vi "NanotecSMCPD.i attribute.vi"(0 "VI Refnum":refnum<vi>, 2 "CLASS.i attribute":T1, 3 "Action":T2(ring), 5 "error in (no error)":errorcluster) -> (14 "VI Refnum out":refnum<vi>, 16 "CLASS.i attribute out":T1, 19 "error out":errorcluster)   [LabVIEW 2014, in "NanotecSMCPD.lvlib"]
doc: "This is a so-called functional global variable. It manages the access to a global variable in a thread-safe way. \n\nHere the attribute data of all instances of THIS class are stored. This is done for performance reasons.\n\nThe indicator \"attribute out\" carries only valid data upon calling the function \"get data\"\n\nLicense Agreement for this software:\n\nCopyright (C)\nGesellschaft für Schwerionenforschung, GSI\nPlanckstr. 1\n64291 Darmstadt\nGermany\n\nContact: D.Beck@gsi.de \n\nThis program is free software; you can redistribute it and/or modify it under the terms of the GNU General Public License as published by the Free Software Foundation; either version 2 of the license, or (at your option) any later version.\n\nThis program is distributed in the hope that it will be useful, but WITHOUT ANY WARRANTY; without even the implied warranty of MERCHANTABILITY or FITNESS FOR A PARTICULAR PURPOSE. See the GNU General License for more details (http://www.gnu.org).\n\nGesellschaft für Schwerionenforschung, GSI\nPlanckstr. 1, 64291 Darmstadt, Germany\nFor all questions and ideas contact: M.Richter@gsi.de, H.Brand@gsi.de or D.Beck@gsi.de.\nLast update: 17-JUN-2004"
uses:
  NanotecSMCPD.lvlib
  NanotecSMCPD.i attribute.ctl
  CSCore/CSSystem/CoreDefs/CoreDefs.error_type.ctl
  CSCore/CSSystem/CoreLib/CoreLib.lvlib
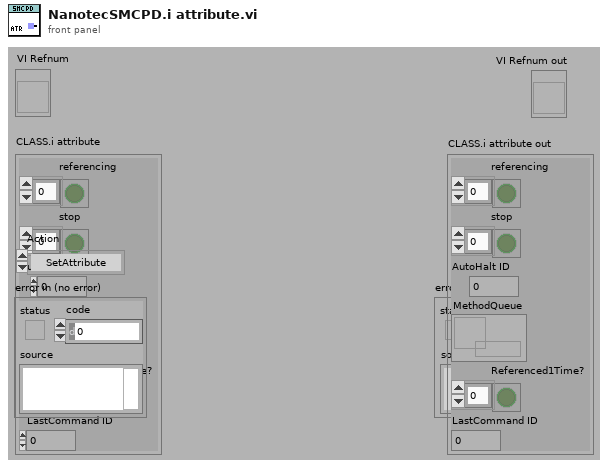
[diagram p1: front panel]
types:
  T1 = typedef "NanotecSMCPD.lvlib/NanotecSMCPD.i attribute.ctl" = cluster{"referencing":bool[], "stop":bool[], "AutoHalt ID":i32, "MethodQueue":refnum<queue>, "Referenced1Time?":bool[], "LastCommand ID":i32}
  T2 = enum16{"SetAttribute", "GetAttribute", "CreateAttribute", "DestroyAttribute", "DestroyAllAtributes"}
  T3 = typedef "CoreDefs.error_type.ctl" = enum16{"no error", "can't load process", "can't unload process", "process does not exist", "can't install process", "can't remove process", "unknown function", "time out", "can't execute function", "duplicate queue name", "super not found", "caller queue invalid", "can't ping process", "unknown error", "VISA Error", "VISA timeout", "GPIB timeout", "GPIB error", "communication error", "data type mismatch", "can't read data from OPC server", "can't write data to OPC server", "OET error", "function not implemented", "process already exists", "invalid Shared Variable name", "error writing Shared Variable", "error reading Shared Variable", "invalid client name", "corrupt database", "unknown class", "call not authorized", "parameter out of range", "OET timeout: can't get data to modify", "invalid queue name", "requested operation incompatible with current state", "event undefined", "event disabled", "state undefined", "caller is not a friend", "EventBuilder: bad eventID", "EventBuilder: no DAQ devices", "a thread must not stop itself", "UNUSED ELEMENT4", "DiscArchiver: eventData incomplete", "DiscArchiver: eventData does not belong to run", "DiscArchiver: can't open file", "DiscArchiver: can't write to file", "DiscArchiver: available disc space low", "can't acquire semaphore", "error reading data from database", "notifier object is not existing", "can't register process", "can't unregister process", "illegal event type", "object disabled", "object already exists", "can't change state", "Instrument not found", "no connection to remote node", "invalid reference", "N/A", "UNUSED ELEMENT 1", "element not found", "illegal TCP/IP connection detected", "object does not exist", "invalid access ID", "unknown CS system", "invalid privilige", "unsupported data type", "unsupported server type", "IO server already exists", "Shared Variable already exists"}
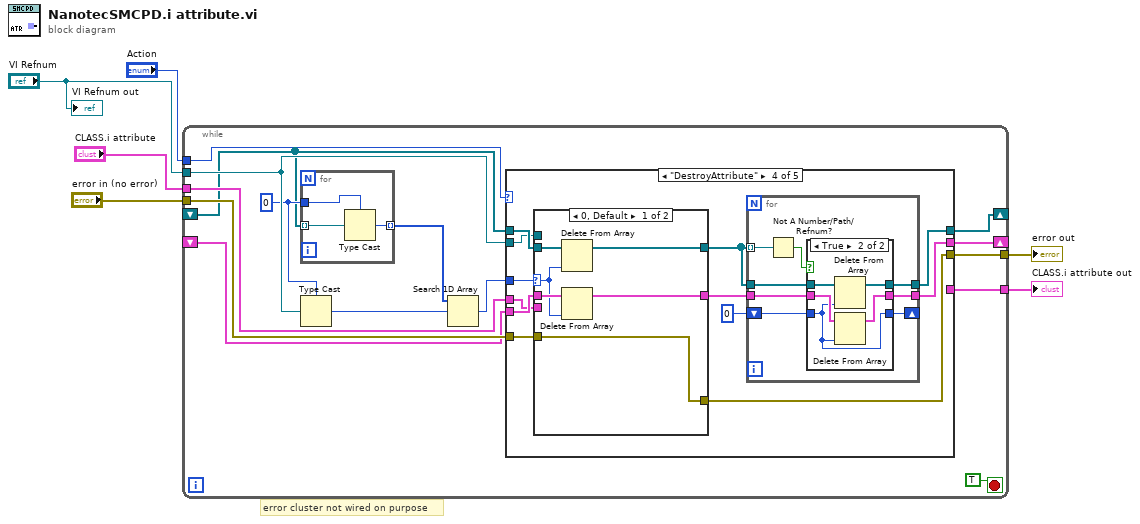
[diagram p0: block diagram]
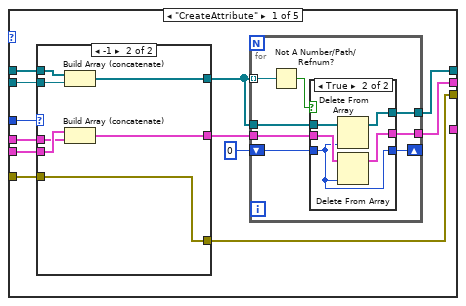
[diagram p2: hidden frame]
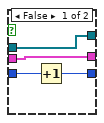
[diagram p3: hidden frame]
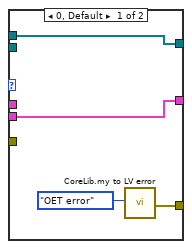
[diagram p4: hidden frame]
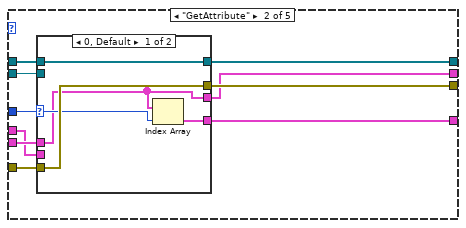
[diagram p5: hidden frame]
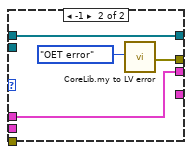
[diagram p6: hidden frame]
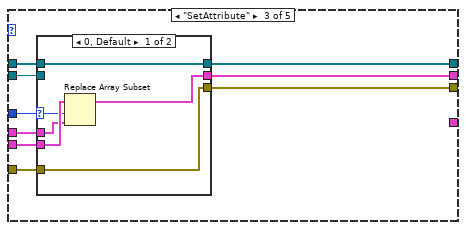
[diagram p7: hidden frame]
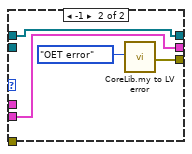
[diagram p8: hidden frame]
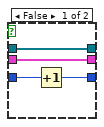
[diagram p9: hidden frame]
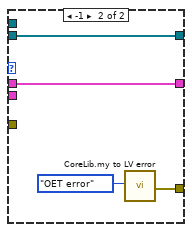
[diagram p10: hidden frame]
diagram:
  # "error cluster not wired on purpose"
  n1 = while {
    shift-right: [w15] -> _
    shift-left: _ -> [w16]
    tunnel: "Action" -> [w20]
    shift-right: [w17] -> _
    shift-left: _ -> [w7]
    tunnel: "error in (no error)" -> [w19]
    tunnel: [w18] -> w4
    tunnel: "CLASS.i attribute" -> [w14]
    tunnel: [w12] -> w2
    tunnel: "VI Refnum" -> [w10]
    stop <- TRUE stop-if-true
    w9 = 0
    n2 = for {
      tunnel: w9 -> [w24]
      tunnel: [w23] -> w8 mode=indexing
      tunnel: w7 -> [w22] mode=indexing
      n3 = Type Cast(type=w24, x=w22) -> (*(type *) &x=w23:i32)
    }
    n4 = Type Cast(type=w9, x=w10) -> (*(type *) &x=w11:i32)
    n5 = Search 1D Array(1D array=w8, element=w11) -> (index of element=w13:i32)  [unwired: 1 in]
    n6 = case shown="\"DestroyAttribute\"" w20 {
      tunnel: w7 -> [w34 w72 w90 w112 _]
      tunnel: w10 -> [w33 w70 w88 w111 _]
      tunnel: w19 -> [w36 w74 w92 w114 w142]
      tunnel: [w35 w73 w91 w113 w142] -> w18
      tunnel: [w28 w71 w89 w106 _] -> w17
      tunnel: w16 -> [w32 w69 w87 w110 _]
      tunnel: [w27 w68 w86 w104 _] -> w15
      tunnel: w14 -> [w31 w67 w85 w109 _]
      tunnel: w13 -> [w30 w66 w84 w108 _]
      tunnel: [_ w65 _ _ _] -> w12
      frame "CreateAttribute" {
        n7 = case shown="-1" w30 {
          tunnel: w36 -> [_ w64]
          tunnel: [w56 w64] -> w35
          tunnel: w34 -> [w55 w63]
          tunnel: [w55 w62] -> w26
          tunnel: w33 -> [_ w61]
          tunnel: w32 -> [w54 w60]
          tunnel: [w54 w59] -> w25
          tunnel: w31 -> [_ w58]
          frame 0, Default {
            n8 = call "CoreLib.my to LV error.vi"("ErrorTypes"=CoreDefs.error_type."OET error") -> ("myErrorCluster"=w56:errorcluster)  [unwired: 17 in, 1 out]
          }
          frame -1 {
            n9 = Build Array (concatenate)(w63, w61) -> (w62:refnum<vi>[])
            n10 = Build Array (concatenate)(w60, w58) -> (w59:T1[])
          }
        }
        n11 = for {
          tunnel: w26 -> [w41]
          tunnel: [w40] -> w28
          tunnel: [w44] -> w27
          tunnel: w25 -> [w43]
          tunnel: w26 -> [w39] mode=indexing
          shift-right: [w38] -> _
          shift-left: 0 -> [w37]
          n12 = Not A Number/Path/Refnum?(number/path/refnum=w39) -> (NaN/Path/Refnum?=w42:bool)
          n13 = case shown="True" w42 {
            tunnel: [w48 w53] -> w44
            tunnel: w43 -> [w48 w52]
            tunnel: [w47 w50] -> w40
            tunnel: w41 -> [w47 w51]
            tunnel: w37 -> [w46 w49]
            tunnel: [w45 w49] -> w38
            frame False {
              n14 = Increment(x=w46) -> (x+1=w45:i32)
            }
            frame True {
              n15 = Delete From Array(array=w51, index=w49) -> (array with subset deleted=w50:refnum<vi>[])  [unwired: 1 in, 1 out]
              n16 = Delete From Array(array=w52, index=w49) -> (array with subset deleted=w53:T1[])  [unwired: 1 in, 1 out]
            }
          }
        }
      }
      frame "GetAttribute" {
        n17 = case shown="0, Default" w66 {
          selector: w66 -> [w77 _]
          tunnel: w74 -> [w79 _]
          tunnel: [w79 w82] -> w73
          tunnel: w72 -> [w78 w81]
          tunnel: [w78 w81] -> w71
          tunnel: w70 -> [_ _]
          tunnel: w69 -> [w76 w80]
          tunnel: [w76 w80] -> w68
          tunnel: w67 -> [_ _]
          tunnel: [w75 _] -> w65
          frame 0, Default {
            n18 = Index Array(array=w76, index=w77) -> (element=w75:T1)
          }
          frame -1 {
            n19 = call "CoreLib.my to LV error.vi"("ErrorTypes"=CoreDefs.error_type."OET error") -> ("myErrorCluster"=w82:errorcluster)  [unwired: 17 in, 1 out]
          }
        }
      }
      frame "SetAttribute" {
        n20 = case shown="0, Default" w84 {
          selector: w84 -> [w94 _]
          tunnel: w92 -> [w98 _]
          tunnel: [w98 w101] -> w91
          tunnel: w90 -> [w97 w100]
          tunnel: [w97 w100] -> w89
          tunnel: w88 -> [_ _]
          tunnel: w87 -> [w96 w99]
          tunnel: [w95 w99] -> w86
          tunnel: w85 -> [w93 _]
          frame 0, Default {
            n21 = Replace Array Subset(array=w96, new element=w93, index=w94) -> (w95:T1[])
          }
          frame -1 {
            n22 = call "CoreLib.my to LV error.vi"("ErrorTypes"=CoreDefs.error_type."OET error") -> ("myErrorCluster"=w101:errorcluster)  [unwired: 17 in, 1 out]
          }
        }
      }
      frame "DestroyAttribute" {
        n23 = case shown="0, Default" w108 {
          selector: w108 -> [w133 _]
          tunnel: w114 -> [w137 _]
          tunnel: [w137 w140] -> w113
          tunnel: w112 -> [w136 w139]
          tunnel: [w135 w139] -> w105
          tunnel: w111 -> [_ _]
          tunnel: w110 -> [w134 w138]
          tunnel: [w132 w138] -> w103
          tunnel: w109 -> [_ _]
          frame 0, Default {
            n24 = Delete From Array(array=w136, index=w133) -> (array with subset deleted=w135:refnum<vi>[])  [unwired: 1 in, 1 out]
            n25 = Delete From Array(array=w134, index=w133) -> (array with subset deleted=w132:T1[])  [unwired: 1 in, 1 out]
          }
          frame -1 {
            n26 = call "CoreLib.my to LV error.vi"("ErrorTypes"=CoreDefs.error_type."OET error") -> ("myErrorCluster"=w140:errorcluster)  [unwired: 17 in, 1 out]
          }
        }
        n27 = for {
          tunnel: w105 -> [w119]
          tunnel: [w118] -> w106
          tunnel: [w122] -> w104
          tunnel: w103 -> [w121]
          tunnel: w105 -> [w117] mode=indexing
          shift-right: [w116] -> _
          shift-left: 0 -> [w115]
          n28 = Not A Number/Path/Refnum?(number/path/refnum=w117) -> (NaN/Path/Refnum?=w120:bool)
          n29 = case shown="True" w120 {
            tunnel: [w126 w131] -> w122
            tunnel: w121 -> [w126 w130]
            tunnel: [w125 w128] -> w118
            tunnel: w119 -> [w125 w129]
            tunnel: w115 -> [w124 w127]
            tunnel: [w123 w127] -> w116
            frame False {
              n30 = Increment(x=w124) -> (x+1=w123:i32)
            }
            frame True {
              n31 = Delete From Array(array=w129, index=w127) -> (array with subset deleted=w128:refnum<vi>[])  [unwired: 1 in, 1 out]
              n32 = Delete From Array(array=w130, index=w127) -> (array with subset deleted=w131:T1[])  [unwired: 1 in, 1 out]
            }
          }
        }
      }
      frame "DestroyAllAtributes" {
      }
    }
  }
  "error out" <- w4
  "CLASS.i attribute out" <- w2
  "VI Refnum out" <- "VI Refnum"
